vi "Noise-Generator.vi"() -> ()   [LabVIEW 2020]
uses:
  <vilib>/Analysis/2dsp.llb/Real FFT.vi
  <vilib>/Analysis/1siggen.llb/Halton Sequence.vi
  <vilib>/Analysis/NI_AALPro.lvlib
  <vilib>/Analysis/NI_AALBase.lvlib
  <vilib>/Analysis/NI_AAL_SignalGeneration.lvlib
panel:
  out "FFT":dbl[](graph)
  in  "dt":dbl=0.1
  in  "Delay":i32=50
  in  "SigFrequency":dbl=1.0 format="%.2f"
  in  "Samples":i32=256
  in  "Duration":dbl=1.0 format="%0.2f"
  in  "dc offset":dbl format="%0.2f"
  in  "Phase":dbl format="%0.2f"
  in  "Amplitude":dbl=1.0 format="%.2f"
  in  "Tab":T1(tab)
  out "Graph":dbl[](graph)
  out "Error":i32
  out "Phase out":dbl format="%.2f"
  # "Noise Generator"
  # "Instruction:\n1) Select signal from tab;\n2) Set parameters of selected signals;\n3) Run VI and check out the wave and frequency of the signal;\n4) Repeat step 1-3 to see other signal."
  # "Common Parameters"
  # "Hz"
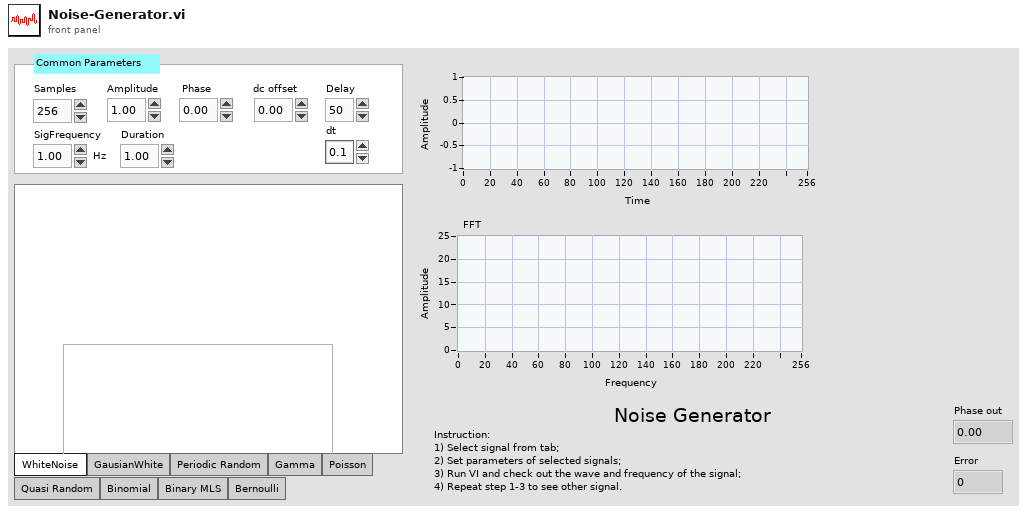
[diagram p1: front panel]
types:
  T1 = enum32{"WhiteNoise ", "GausianWhite", "Periodic Random", "Gamma", "Poisson", "Quasi Random", "Binomial", "Binary MLS", "Bernoulli"}
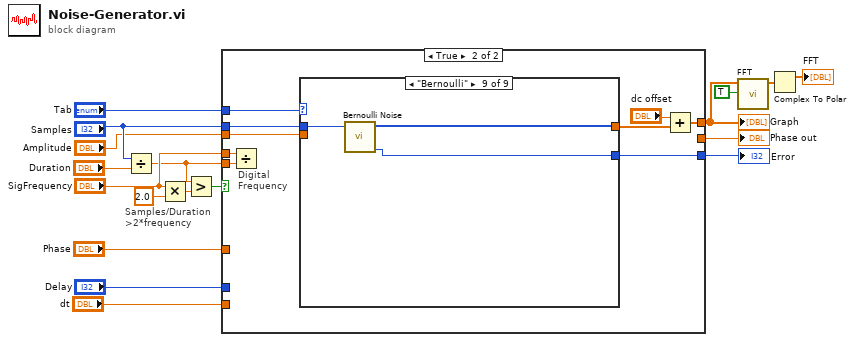
[diagram p0: block diagram]
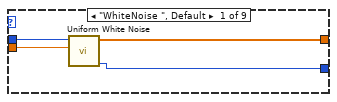
[diagram p3: hidden frame]
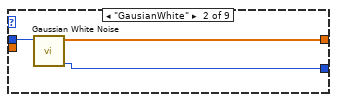
[diagram p4: hidden frame]
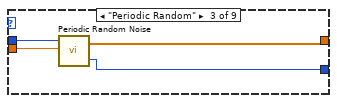
[diagram p5: hidden frame]
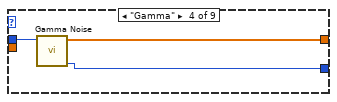
[diagram p6: hidden frame]
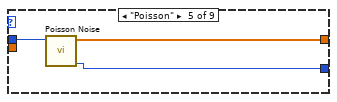
[diagram p7: hidden frame]
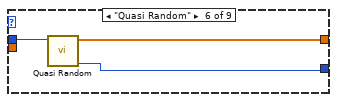
[diagram p8: hidden frame]
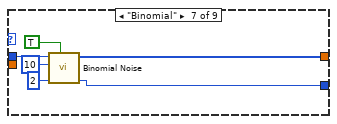
[diagram p9: hidden frame]
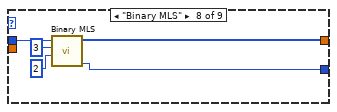
[diagram p10: hidden frame]
diagram:
  # "Samples/Duration \n>2*frequency"
  n1 = Divide(x="Samples", y="Duration") -> (x/y=w8:dbl)
  n2 = Multiply(x="SigFrequency", y=2.0) -> (x*y=w7:dbl)
  n3 = Greater?(x=w8, y=w7) -> (0:w11:bool)
  n4 = case shown="True" w11 {
    tunnel: w8 -> [_ w30]
    tunnel: "Samples" -> [_ w25]
    tunnel: "SigFrequency" -> [_ w28]
    tunnel: [-20061 ("error") w22] -> w18
    tunnel: [dbl[] [] ("Signal") w26] -> w4
    tunnel: "Tab" -> [_ w27]
    tunnel: "Amplitude" -> [_ w24]
    tunnel: "Phase" -> [w19 _]
    tunnel: [w19 _] -> w12
    tunnel: "Delay" -> [_ _]
    tunnel: "dt" -> [_ _]
    frame False {
      # "Error: Nyquist Criterion violated\nsamples/duration must be > 2*frequency\nYou must adjust samples, duration, or frequency by:\n     increasing #samples\n     decreasing duration\n     decreasing frequency"
    }
    frame True {
      # "Digital \nFrequency"
      n5 = Divide(x=w28, y=w30) -> ()  [unwired: 1 out]
      n6 = case shown="\"Bernoulli\"" w27 {
        tunnel: w25 -> [w34 w37 w41 w44 w47 w50 w56 w61 w64]
        tunnel: w24 -> [w33 _ w40 _ _ _ _ _ _]
        tunnel: [w32 w36 w39 w43 w45 w48 w55 w59 w62] -> w23
        tunnel: [w31 w35 w38 w42 w46 w49 w54 w60 w63] -> w22
        frame "WhiteNoise ", Default {
          n7 = call <vilib>:"Uniform White Noise.vi"("amplitude"=w33, "samples"=w34) -> ("error"=w31:i32, "uniform white noise"=w32:dbl[])  [unwired: 8 in]
        }
        frame "GausianWhite" {
          n8 = call <vilib>:"Gaussian White Noise.vi"("samples"=w37) -> ("error"=w35:i32, "Gaussian noise pattern"=w36:dbl[])  [unwired: 9 in]
        }
        frame "Periodic Random" {
          n9 = call <vilib>:"Periodic Random Noise.vi"("spectral amplitude"=w40, "samples"=w41) -> ("error"=w38:i32, "periodic random noise"=w39:dbl[])  [unwired: 1 in]
        }
        frame "Gamma" {
          n10 = call <vilib>:"Gamma Noise.vi"("samples"=w44) -> ("error"=w42:i32, "gamma noise"=w43:dbl[])  [unwired: 9 in]
        }
        frame "Poisson" {
          n11 = call <vilib>:"Poisson Noise.vi"("samples"=w47) -> ("error"=w46:i32, "poisson noise"=w45:dbl[])  [unwired: 9 in]
        }
        frame "Quasi Random" {
          n12 = call-poly <vilib>:"Quasi Random.vi"("samples"=w50) -> ("error"=w49:i32, "Halton Pattern"=w48:dbl[])  [unwired: 9 in]
        }
        frame "Binomial" {
          n13 = call <vilib>:"Binomial Noise.vi"("initialize?"=TRUE, "seed"=2, "trials"=10, "samples"=w56) -> ("error"=w54:i32, "binomial noise"=w55:u32[])  [unwired: 6 in]
        }
        frame "Binary MLS" {
          n14 = call <vilib>:"Binary MLS.vi"("seed"=i64 2, "polynomial order"=3, "samples"=w61) -> ("error code"=w60:i32, "mls sequence"=w59:u8[])  [unwired: 7 in]
        }
        frame "Bernoulli" {
          n15 = call <vilib>:"Bernoulli Noise.vi"("samples"=w64) -> ("error"=w63:i32, "bernoulli noise"=w62:u8[])  [unwired: 9 in]
        }
      }
      n16 = Add(x="dc offset", y=w23) -> (x+y=w26:dbl[])
    }
  }
  "Error" <- w18
  "Graph" <- w4
  "Phase out" <- w12
  n17 = call-poly <vilib>:"FFT.vi"("shift?"=TRUE, "X"=w4) -> ("FFT {X}"=w3:cdb[])  [unwired: 8 in, 1 out]
  n18 = Complex To Polar(r * e^(i*theta)=w3) -> (r=→"FFT":dbl[])  [unwired: 1 out]
